vi "ActionVIOnLoad - Version.vi"(8 "error in (no error)":errorcluster, 11 "Device Item Ref in":T1 format="%.0x") -> (0 "error out":errorcluster, 3 "Device Item Ref out":T1 format="%.0x")   [LabVIEW 2019, in "Instrument Addon System Explorer.lvlib"]
uses:
  Instrument Addon System Explorer.lvlib
  <vilib>/NI VeriStand/Custom Device API/Custom Device Item Ref.ctl
  NationalInstruments.VeriStand.SystemDefinitionAPI
  Shared/Constants.vi
  <vilib>/NI VeriStand/Custom Device API/Custom Device API.lvlib
  Shared/Instrument Addon Shared.lvlib
  <vilib>/NI VeriStand/Custom Device Tools/Custom Device Utility Library/Custom Device Utility Library.lvlib
  <vilib>/NI VeriStand/Custom Device Tools/Custom Device Utility Library/NI VeriStand - Search for All Items by GUID.vi
  <vilib>/NI VeriStand/Custom Device API/Custom Device Channel Type.ctl
  <vilib>/NI VeriStand/Custom Device API/Custom Device Channel.ctl
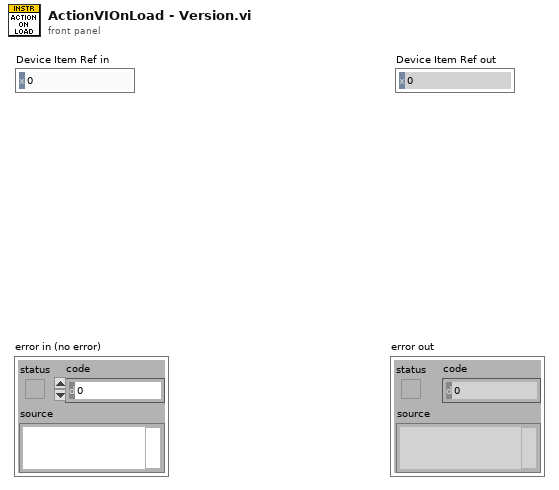
[diagram p1: front panel]
types:
  T1 = typedef "Custom Device API.lvlib/Custom Device Item Ref.ctl" = u64
  T2 = typedef "Custom Device API.lvlib/Custom Device Channel.ctl" = cluster{"Type":T3, "Units":string, "Default Value":dbl, "Faultable":bool, "Scalable":bool}
  T3 = typedef "Custom Device API.lvlib/Custom Device Channel Type.ctl" = enum16{"Input", "Output"}
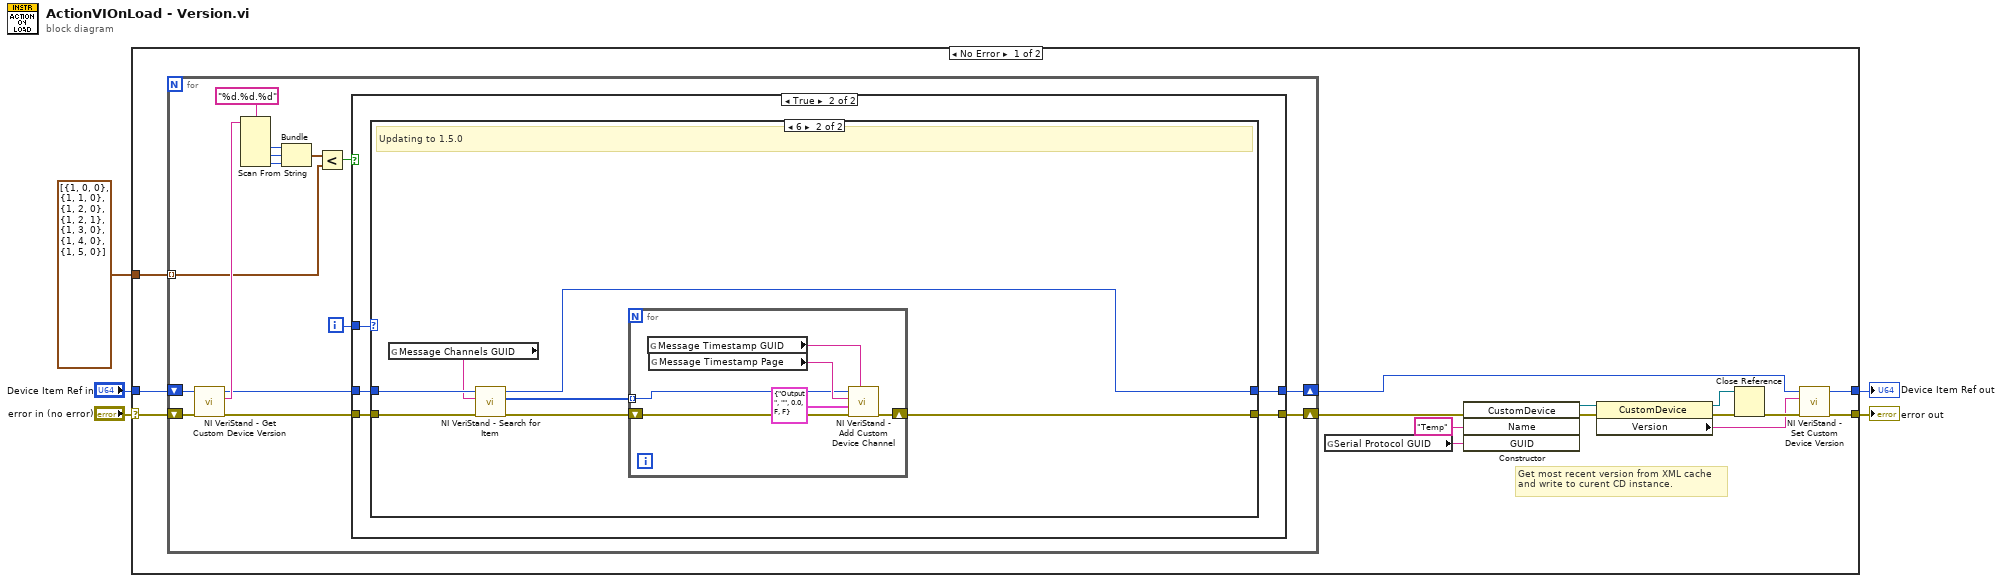
[diagram p0: block diagram]
diagram:
  n1 = case shown="No Error" "error in (no error)" {
    selector: "error in (no error)" -> [w20 w59]
    tunnel: [w10 w59] -> w2
    tunnel: "Device Item Ref in" -> [w19 w58]
    tunnel: [w11 w58] -> w1
    tunnel: cluster{i32, i32, i32}[] [{1, 0, 0}, {1, 1, 0}, {1, 2, 0}, {1, 2, 1}, {1, 3, 0}, {1, 4, 0}, {1, 5, 0}] -> [w18 _]
    frame No Error {
      # "Get most recent version from XML cache\nand write to curent CD instance."
      n2 = for {
        shift-right: [w26] -> w9
        shift-left: w20 -> [w31]
        shift-right: [w24] -> w8
        shift-left: w19 -> [w30]
        tunnel: w18 -> [w21] mode=indexing
        i -> [w23]
        n3 = call <vilib>:"NI VeriStand - Get Custom Device Version.vi"("error in (no error)"=w31, "Device Ref in"=w30) -> ("error out"=w27:errorcluster, "Value"=w29:string, "Device Ref out"=w25:T1)  [unwired: 7 in]
        n4 = Scan From String(format string="%d.%d.%d", input string=w29) -> (output 1=w33:i32, output 2=w34:i32, output 3=w22:i32)  [unwired: 5 in, 3 out]
        n5 = Bundle(w33, w34, w22) -> (w35:cluster{i32, i32, i32})  [unwired: 1 in]
        n6 = Less?(x=w35, y=w21) -> (x < y?=w28:bool)
        n7 = case shown="True" w28 {
          tunnel: w27 -> [w37 w42]
          tunnel: [w37 w41] -> w26
          tunnel: w25 -> [w36 w38]
          tunnel: [w36 w39] -> w24
          tunnel: w23 -> [_ w40]
          frame False {
          }
          frame True {
            n8 = case shown="6" w40 {
              tunnel: w42 -> [w44 w50]
              tunnel: [w44 w45] -> w41
              tunnel: [w43 w46] -> w39
              tunnel: w38 -> [w43 w51]
              frame Default {
              }
              frame 6 {
                # "Updating to 1.5.0"
                n9 = global read "Constants.vi" "Message Channels GUID"() -> (w49:string)
                n10 = call-poly <vilib>:"NI VeriStand - Search for Item.vi"("error in"=w50, "Item GUID"=w49, "Section Ref in"=w51) -> ("error out"=w48:errorcluster, "Item Refs"=w47:T1[], "Section Ref out"=w46:T1)  [unwired: 5 in, 1 out]
                n11 = for {
                  tunnel: w47 -> [w52] mode=indexing
                  shift-right: [w53] -> w45
                  shift-left: w48 -> [w54]
                  n12 = global read "Constants.vi" "Message Timestamp GUID"() -> (w56:string)
                  n13 = global read "Constants.vi" "Message Timestamp Page"() -> (w57:string)
                  n14 = call <vilib>:"NI VeriStand - Add Custom Device Channel.vi"("GUID (Default Channel)"=w56, "error in (no error)"=w54, "Channel"=T2 {"Type"=enum."Output", "Units"="", "Default Value"=0.0, "Faultable"=FALSE, "Scalable"=FALSE}, "Channel Name"=w57, "Parent Ref in"=w52) -> ("error out"=w53:errorcluster)  [unwired: 3 in, 3 out]
                }
              }
            }
          }
        }
      }
      n15 = global read "Constants.vi" "Serial Protocol GUID"() -> (w6:string)
      n16 = constructor class="CustomDevice"(error in=w9, "Name"="Temp", "GUID"=w6) -> (reference out=w17:refnum<k24>, error out=w16:errorcluster)  [unwired: 2 in, 3 out]
      n17 = property class="CustomDevice"(reference=w17, error in=w16) -> (reference out=w14:refnum<k24>, error out=w15:errorcluster, "Version"=w12:string)
      n18 = Close Reference(reference=w14, error in (no error)=w15) -> (error out=w13:errorcluster)
      n19 = call <vilib>:"NI VeriStand - Set Custom Device Version.vi"("error in (no error)"=w13, "Value"=w12, "Device Ref in"=w8) -> ("error out"=w10:errorcluster, "Device Ref out"=w11:T1)  [unwired: 7 in]
    }
    frame Error {
    }
  }
  "error out" <- w2
  "Device Item Ref out" <- w1
